vi "Boolean.vi"(4 "true string (1)":string="1", 6 "false string (0)":string="0", 7 "key description":string, 8 "sections":string[](array[string]), 9 "boolean":bool, 11 "info data":string) -> (0 "sections out":string[](array[string]), 3 "info data out":string)   [LabVIEW 2019, in "infolib.lvlib"]
doc: "Add a new boolean key to Info Data string. If section exists in Info Data string, inserts key into this section. If true and false strings are not set, boolean is represented as \"1\" or \"0\"."
uses:
  infolib.lvlib
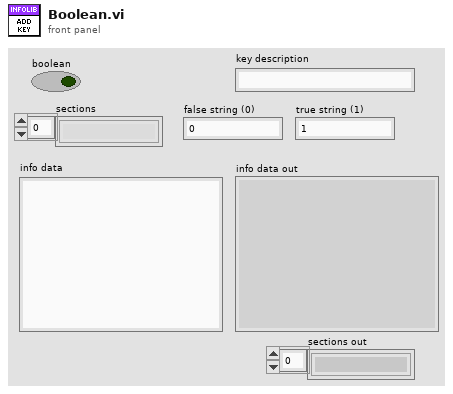
[diagram p1: front panel]
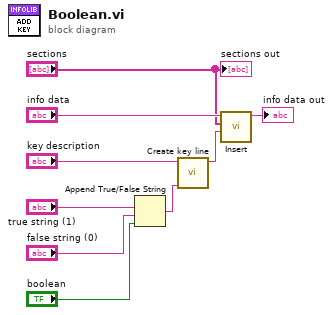
[diagram p0: block diagram]
diagram:
  n1 = Append True/False String(1:"boolean", 2:"false string (0)", 3:"true string (1)") -> (0:w6:string)  [unwired: 1 in]
  n2 = call "Create key line.vi"("formatted value"=w6, "key description"="key description") -> ("line"=w1:string)  [unwired: 9 in]
  n3 = call "Insert.vi"("insert"=w1, "sections"="sections", "info data"="info data") -> ("info data out"=→"info data out":string)  [unwired: 8 in]
  "sections out" <- "sections"
